vi "Handle INVOCATION.vi"(8 "error in (no error)":errorcluster, 9 "Message Loop Shift Register Data":T1, 10 "Cluster":T15 {"Message Codes" items=["HELLO"=1, "WELCOME"=2, "ABORT"=3, "GOODBYE"=6, "ERROR"=8, "PUBLISH"=16, "PUBLISHED"=17, "SUBSCRIBE"=32, "SUBSCRIBED"=33, "UNSUBSCRIBE"=34, "UNSUBSCRIBED"=35, "EVENT"=36, "CALL"=48, "RESULT"=59, "REGISTER"=64, "REGISTERED"=65, "UNREGISTER"=66, "UNREGISTERED"=67, "INVOCATION"=68, "YIELD"=70]}, 11 "reference":refnum<class "WAMP Client.lvclass">) -> (0 "error out":errorcluster, 3 "reference out":refnum<class "WAMP Client.lvclass">)   [LabVIEW 2020, in "wamplv.lvlib" / "WAMP Client.lvclass"]
uses:
  WAMP Client.lvclass
  WAMP Client.lvclass/WAMP Client.ctl
  API/TypeDefs/INVOCATION payload.ctl
  Private/Invocation Request ID/Invocation Request ID.lvclass
  Private/TypeDefs/WAMP Message Codes.ctl
  wamplv.lvlib
  TypeDef/WAMP Received Message.ctl
  API/TypeDefs/WAMP error.ctl
  TypeDef/Success or error.ctl
  TypeDef/REGISTER Request Data.ctl
  TypeDef/PUBLISH Request Data.ctl
  TypeDef/Publish Requests Map.ctl
  TypeDef/Endpoint Data.ctl
  TypeDef/Message Loop Data.ctl
  TypeDef/CALL Request Map.ctl
  TypeDef/EVENT payload.ctl
  TypeDef/Subscribe Result.ctl
  TypeDef/SUBSCRIBE Request Data.ctl
  TypeDef/SUBSCRIBE Requests Map.ctl
  TypeDef/Subscription Details.ctl
  TypeDef/Subscriptions Map.ctl
  TypeDef/UNSUBSCRIBE Result.ctl
  TypeDef/UNSUBSCRIBE Request Data.ctl
  TypeDef/Unsubscribe Requests Map.ctl
  API/TypeDefs/Combined error.ctl
  TypeDef/Unregister request.ctl
  TypeDef/Unregister requests map.ctl
  TypeDef/PUBLISH result.ctl
  Private/Requests/ICallRequest/ICallRequest.lvclass
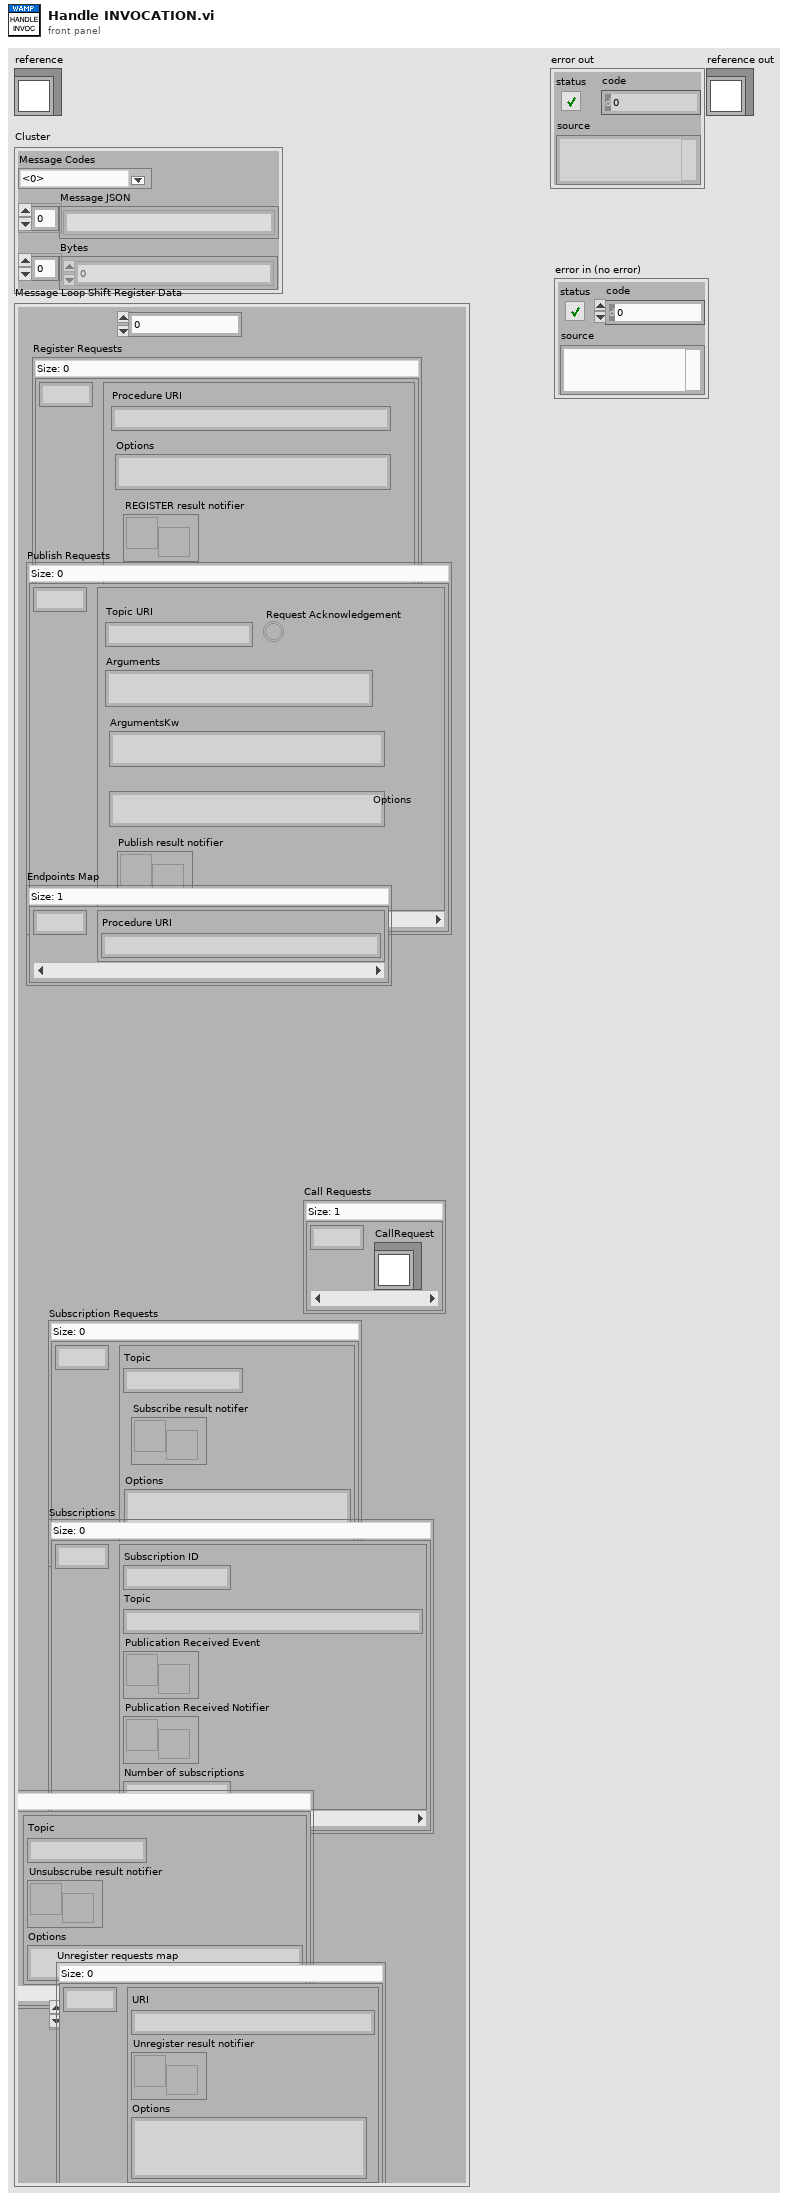
[diagram p1: front panel]
types:
  T1 = typedef "wamplv.lvlib/WAMP Client.lvclass/Message Loop Data.ctl" = cluster{"Last Request ID":u64, "Register Requests":map{u64, T2}, "Publish Requests":T3, "Endpoints Map":map{u64, T5}, "Call Requests":T6, "Subscription Requests":T7, "Subscriptions":T9, "Unsubscribe Requests":T11, "Random Request IDs":u64[], "Unregister requests map":T13}
  T2 = typedef "wamplv.lvlib/WAMP Client.lvclass/REGISTER Request Data.ctl" = cluster{"Procedure URI":string, "Options":string, "REGISTER result notifier":refnum<notifier>}
  T3 = typedef "wamplv.lvlib/WAMP Client.lvclass/Publish Requests Map.ctl" = map{u64, T4}
  T4 = typedef "wamplv.lvlib/WAMP Client.lvclass/PUBLISH Request Data.ctl" = cluster{"Topic URI":string, "Arguments":string, "ArgumentsKw":string, "Request Acknowledgement":bool, "Options":string, "Publish result notifier":refnum<notifier>}
  T5 = typedef "wamplv.lvlib/WAMP Client.lvclass/Endpoint Data.ctl" = cluster{"Procedure URI":string}
  T6 = typedef "wamplv.lvlib/WAMP Client.lvclass/CALL Request Map.ctl" = map{u64, refnum<class "ICallRequest.lvclass">}
  T7 = typedef "wamplv.lvlib/WAMP Client.lvclass/SUBSCRIBE Requests Map.ctl" = map{u64, T8}
  T8 = typedef "wamplv.lvlib/WAMP Client.lvclass/SUBSCRIBE Request Data.ctl" = cluster{"Topic":string, "Subscribe result notifer":refnum<notifier>, "Options":string}
  T9 = typedef "wamplv.lvlib/WAMP Client.lvclass/Subscriptions Map.ctl" = map{u64, T10}
  T10 = typedef "wamplv.lvlib/WAMP Client.lvclass/Subscription Details.ctl" = cluster{"Subscription ID":u64, "Topic":string, "Publication Received Event":refnum<user-event>, "Publication Received Notifier":refnum<notifier>, "Number of subscriptions":u64}
  T11 = typedef "wamplv.lvlib/WAMP Client.lvclass/Unsubscribe Requests Map.ctl" = map{u64, T12}
  T12 = typedef "wamplv.lvlib/WAMP Client.lvclass/UNSUBSCRIBE Request Data.ctl" = cluster{"Topic":string, "Unsubscrube result notifier":refnum<notifier>, "Options":string}
  T13 = typedef "wamplv.lvlib/WAMP Client.lvclass/Unregister requests map.ctl" = map{u64, T14}
  T14 = typedef "wamplv.lvlib/WAMP Client.lvclass/Unregister request.ctl" = cluster{"URI":string, "Unregister result notifier":refnum<notifier>, "Options":string}
  T15 = typedef "wamplv.lvlib/WAMP Client.lvclass/WAMP Received Message.ctl" = cluster{"Message Codes":T16, "Message JSON":string[], "Bytes":u8[]}
  T16 = typedef "wamplv.lvlib/WAMP Message Codes.ctl" = u16
  T17 = typedef "wamplv.lvlib/WAMP Client.lvclass/INVOCATION payload.ctl" = cluster{"Arguments":string, "ArgumentKw":string, "Procedure URI":string, "Details":string, "Registration ID":u64, "Invocation Request ID":refnum<class "Invocation Request ID.lvclass">}
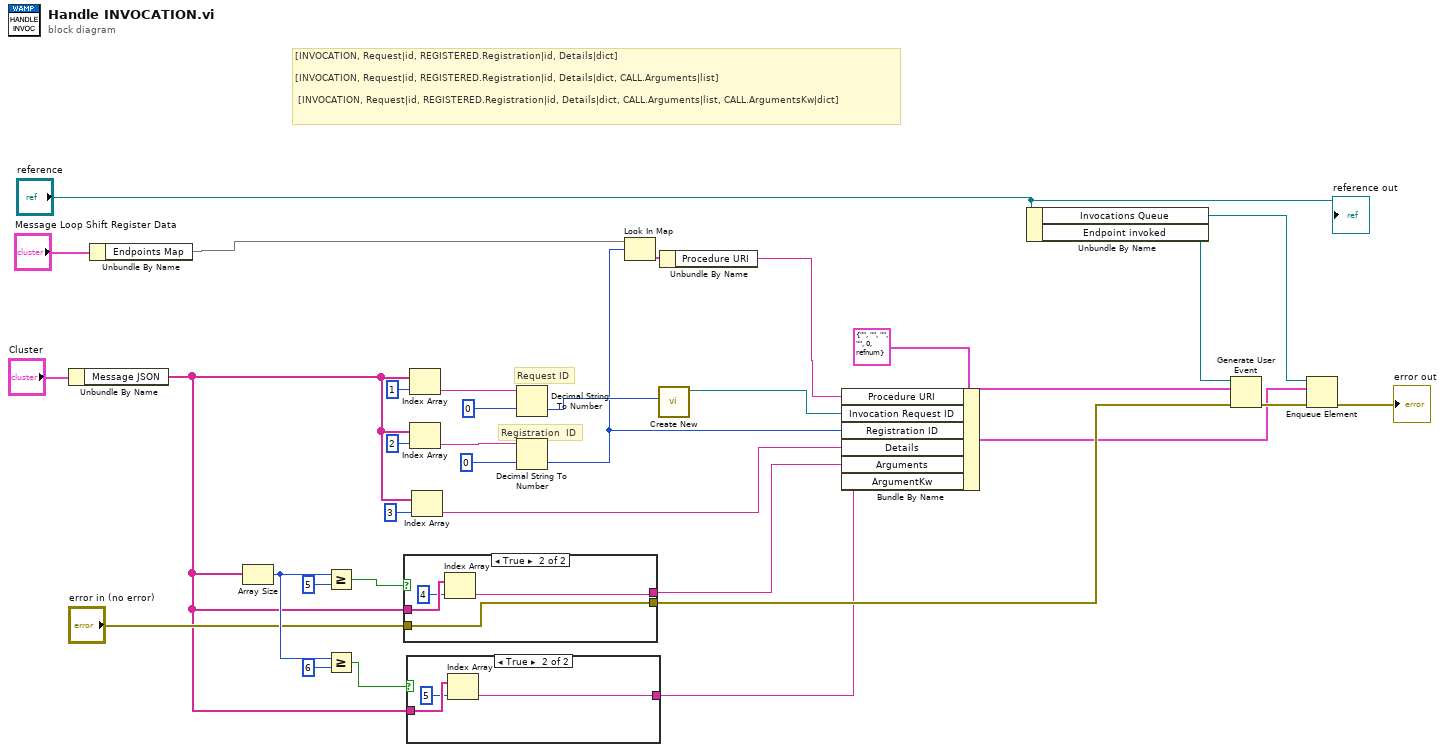
[diagram p0: block diagram]
diagram:
  # "[INVOCATION, Request|id, REGISTERED.Registration|id, Details|dict]\n\n[INVOCATION, Request|id, REGISTERED.Registration|id, Details|dict, CALL.Arguments|list]\n\n [INVOCATION, Request|id, REGISTERED.Registration|id, Details|dict, CALL.Arguments|list, CALL.ArgumentsKw|dict]"
  # "Registration  ID"
  # "Request ID"
  n1 = Unbundle By Name("Cluster") -> ("Message JSON"=w9:string[])
  n2 = Unbundle By Name("Message Loop Shift Register Data") -> ("Endpoints Map"=w13:map{u64, T5})
  n3 = Array Size(array=w9) -> (size(s)=w23:i32)
  n4 = Greater Or Equal?(x=w23, y=5) -> (x >= y?=w25:bool)
  n5 = Greater Or Equal?(x=w23, y=6) -> (x >= y?=w22:bool)
  n6 = case shown="True" w25 {
    tunnel: w9 -> [_ w38]
    tunnel: [_ w35] -> w11
    tunnel: "error in (no error)" -> [w34 w36]
    tunnel: [w34 w36] -> w20
    frame False {
    }
    frame True {
      n7 = Index Array(array=w38, index=4) -> (element=w35:string)
    }
  }
  n8 = case shown="True" w22 {
    tunnel: w9 -> [_ w41]
    tunnel: [_ w39] -> w10
    frame False {
    }
    frame True {
      n9 = Index Array(array=w41, index=5) -> (element=w39:string)
    }
  }
  n10 = Index Array(array=w9, index=1) -> (element=w32:string)
  n11 = Index Array(array=w9, index=2) -> (element=w33:string)
  n12 = Index Array(array=w9, index=3) -> (element=w12:string)
  n13 = Decimal String To Number(string=w32, default (0L)=u64 0) -> (number=w3:u64)  [unwired: 1 in, 1 out]
  n14 = Decimal String To Number(string=w33, default (0L)=u64 0) -> (number=w1:u64)  [unwired: 1 in, 1 out]
  n15 = Look In Map(map=w13, key=w1) -> (value=w18:T5)  [unwired: 1 in, 1 out]
  n16 = call "Create New.vi"("Invocation Request ID"=w3) -> ("Invocation Request out"=w2:refnum<class "Invocation Request ID.lvclass">)  [unwired: 9 in, 1 out]
  n17 = Unbundle By Name(w18) -> ("Procedure URI"=w17:string)
  n18 = Bundle By Name(cluster=T17 {"Arguments"="", "ArgumentKw"="", "Procedure URI"="", "Details"="", "Registration ID"=0, "Invocation Request ID"=refnum} ("INVOCATION payload"), "Procedure URI"=w17, "Invocation Request ID"=w2, "Registration ID"=w1, "Details"=w12, "Arguments"=w11, "ArgumentKw"=w10) -> (w4:T17)
  n19 = Unbundle By Name("reference") -> ("Invocations Queue"=w5:refnum<queue>, "Endpoint invoked"=w15:refnum<user-event>)
  n20 = Generate User Event(user event=w15, event data cluster=w4, error in=w20) -> (error out=w7:errorcluster)  [unwired: 1 in, 1 out]
  n21 = Enqueue Element(queue=w5, element=w4, error in (no error)=w7) -> (error out=→"error out":errorcluster)  [unwired: 1 in, 2 out]
  "reference out" <- "reference"
